vi "Tag FGV.vi"(0 "Operation":T4, 5 "Tag Name":string, 9 "Data":variant, 11 "error in (no error)":errorcluster, 12 "Tag Category":string) -> (2 "Alarm Array":T1[](array[typedef]), 3 "Process Name":string, 4 "Tag Names":string[](array[string]), 6 "Tag Values":dbl[](array[numeric]), 10 "Tag Value":dbl, 13 "Boolean alarm settings":T2, 14 "alarms":T3(array[cluster]) {"value" format="%.2f"; "setpoint" format="%.2f"; "clear time" format="%<%X\n%x>T"; "ack time" format="%<%X\n%x>T"; "set time" format="%<%X\n%x>T"}, 15 "error out":errorcluster)   [LabVIEW 2018, in "Dynamic Shared Variables.lvlib"]
doc: "Handles dynamic tag (shared variable) creation and release as well as alarm configuration and ack."
uses:
  Shared Variables/Dynamic Shared Variables.lvlib
  Tag FGV Operation Enum.ctl
  Numeric Alarm Settings Cluster.ctl
  Utilities/ISO 8601 type.ctl
  Shared Variables/URL Type Enum.ctl
  <vilib>/lvdsc/alarm/Acknowledge Alarms By Instance.vi
  <vilib>/lvdsc/variables/internal/Configure Alarming (Shared Variable, Numeric).vi
  <vilib>/lvdsc/variables/internal/Configure Alarming (Shared Variable, Boolean).vi
  <vilib>/lvdsc/variables/internal/Configure Alarming (Shared Variable, Enable Alarming).vi
  XML Config/XML Config.lvlib
  <vilib>/lvdsc/NI_DSC.lvlib
  <resource>/objmgr/nvio.rc
panel:
  out "Tag Category Array":string[](array[string])
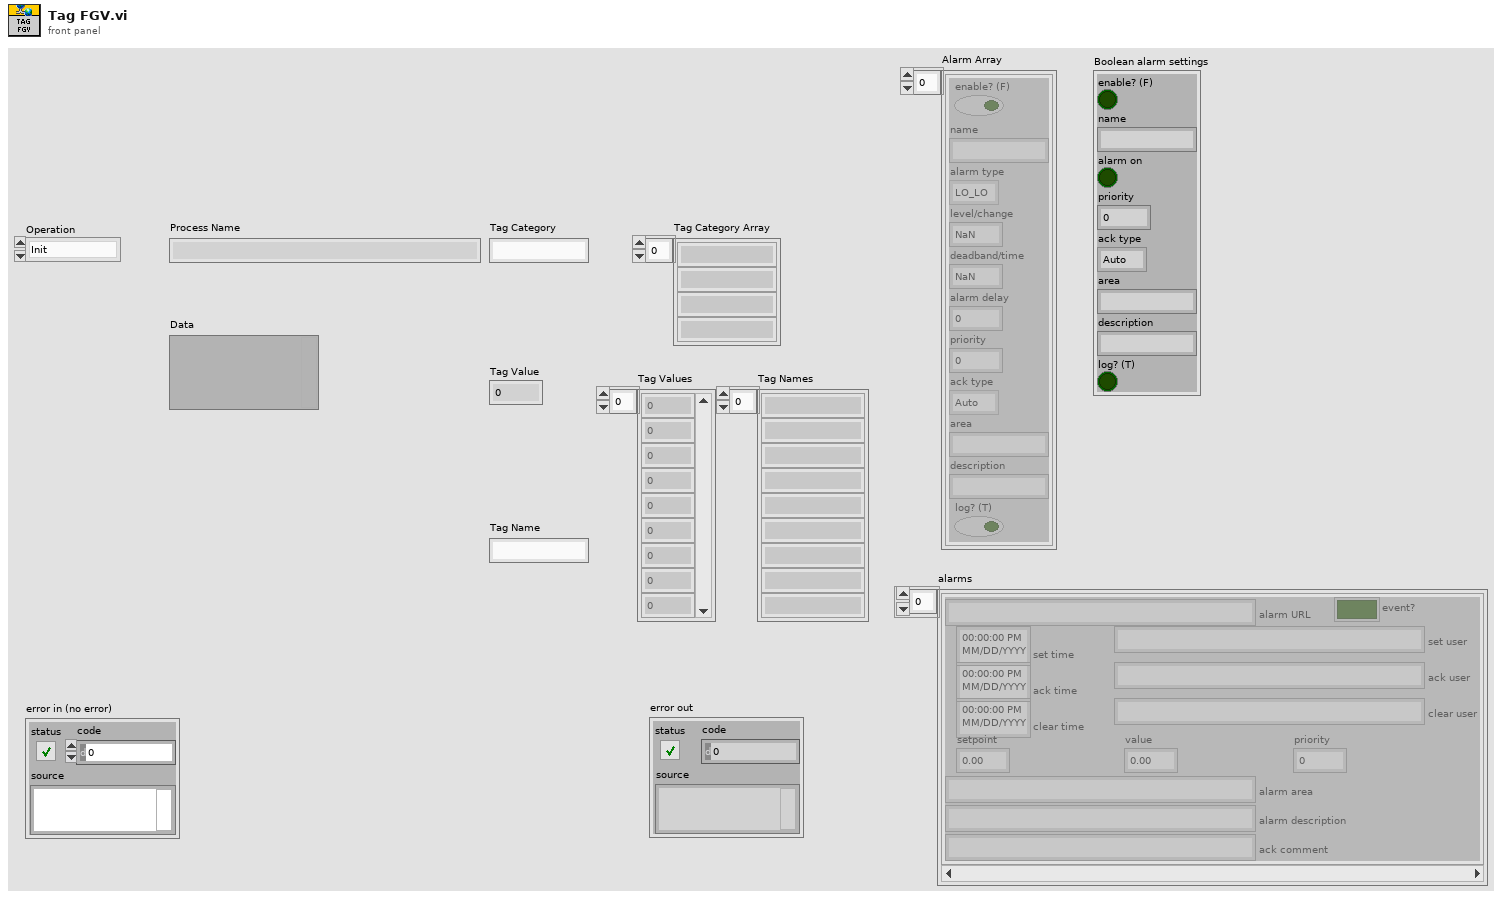
[diagram p1: front panel]
types:
  T1 = typedef "Numeric Alarm Settings Cluster.ctl" = cluster{"enable? (F)":bool, "name":string, "alarm type":enum16{"HI_HI", "HI", "LO", "LO_LO"}, "level/change":dbl, "deadband/time":dbl, "alarm delay":dbl, "priority":u32, "ack type":enum16{"Auto", "User", "None", "Each Occurrence"}, "area":string, "description":string, "log? (T)":bool}
  T2 = cluster{"enable? (F)":bool, "name":string, "alarm on":bool, "priority":u32, "ack type":enum16{"Auto", "User", "None", "Each Occurrence"}, "area":string, "description":string, "log? (T)":bool}
  T3 = cluster{"alarm URL":string, "set time":timestamp, "set user":string, "ack time":timestamp, "ack user":string, "clear time":timestamp, "clear user":string, "setpoint":dbl, "value":dbl, "priority":u32, "alarm area":string, "alarm description":string, "ack comment":string, "event?":bool, "Refnum":u64}[]
  T4 = typedef "Tag FGV Operation Enum.ctl" = enum16{"Init", "Set Notification Queue", "Create Tag", "Commit", "Write Tag (Numeric)", "Write Tag (Boolean)", "Read All Tags", "Read One Tag", "Delete Tag Category", "Set Alarm Parameters (Numeric)", "Set Alarm Parameters (Boolean)", "Enable All Alarms", "Disable All Alarms", "Delete All Tags", "Read Alarms", "Ack Alarm", "Read Alarm Parameters (Numeric)", "Read Alarm Parameters (Boolean)"}
  T5 = typedef "ISO 8601 type.ctl" = enum16{"full ISO 8601 UTC", "basic ISO8601 local", "Windows ISO 8601 UTC", "YYYY-MM-DD UTC", "full ISO 8601 local"}
  T6 = enum32{"u32BitField", "bool", "double", "string", "int8", "uint8", "int16", "uint16", "int32", "uint32", "int64", "uint64", "single", "double waveform", "int16 waveform", "array of boolean", "array of int8", "array of uint8", "array of int16", "array of uint16", "array of int32", "array of uint32", "array of int64", "array of uint64", "array of single", "array of double", "array of double waveform", "array of int16 waveform", "array of string", "variant", "timestamp", "fixed point", "custom"}
  T7 = typedef "Dynamic Shared Variables.lvlib/URL Type Enum.ctl" = enum16{"Tag", "HiHi", "Hi", "Lo", "LoLo", "Tag (Bool)"}
  T8 = cluster{"alarm URL":string, "set time":timestamp, "set user":string, "ack time":timestamp, "ack user":string, "clear time":timestamp, "clear user":string, "setpoint":dbl, "value":dbl, "priority":u32, "alarm area":string, "alarm description":string, "ack comment":string, "event?":bool, "Refnum":u64}
  T9 = enum16{"Auto", "User", "None", "Each Occurrence"}
  T10 = cluster{"enable? (F)":bool, "name":string, "alarm type":enum16{"HI_HI", "HI", "LO", "LO_LO"}, "level/change":dbl, "deadband/time":dbl, "priority":u32, "ack type":enum16{"Auto", "User", "None", "Each Occurrence"}, "area":string, "description":string, "log? (T)":bool}
  T11 = cluster{"enable? (F)":bool, "name":string, "alarm on":bool, "priority":u32, "ack type":enum16{"Auto", "User", "None", "Each Occurrence"}, "area":string, "description":string, "log? (T)":bool}[]
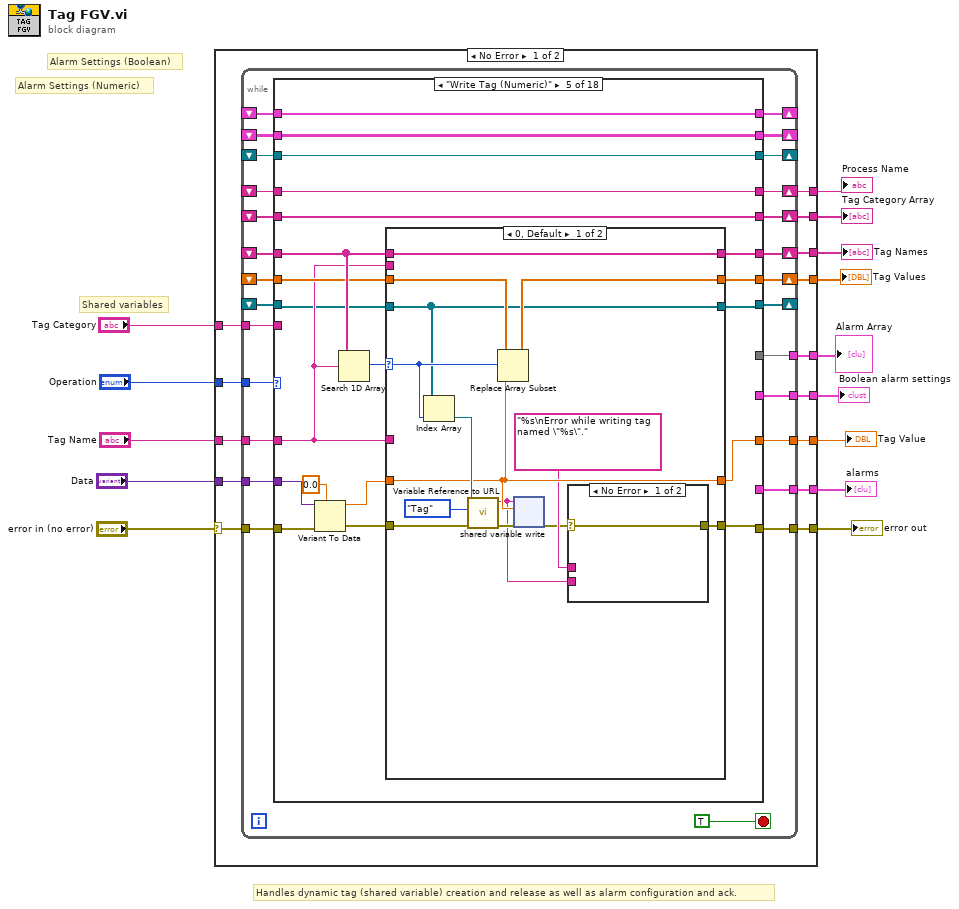
[diagram p0: block diagram]
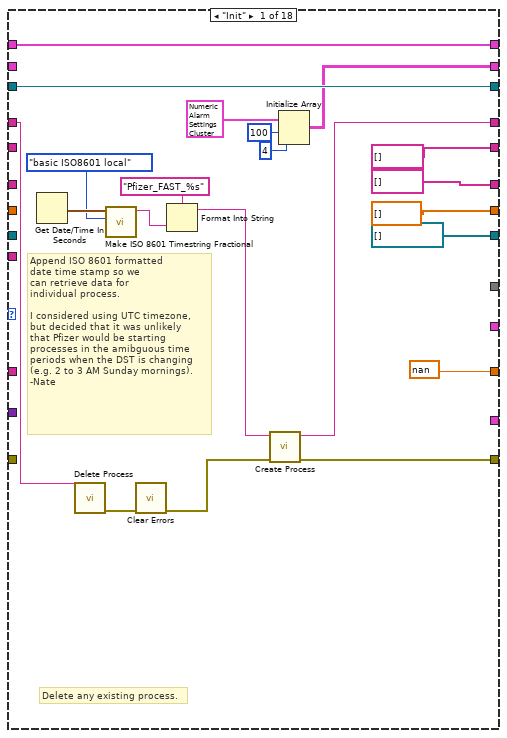
[diagram p2: hidden frame]
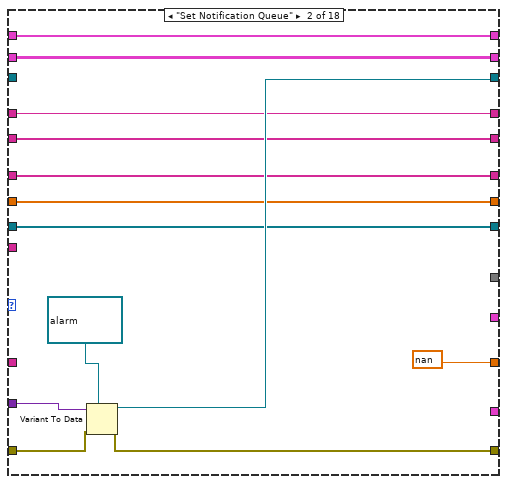
[diagram p3: hidden frame]
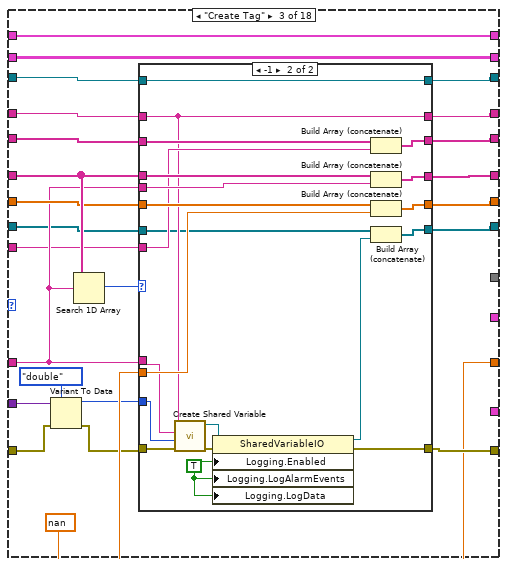
[diagram p4: hidden frame]
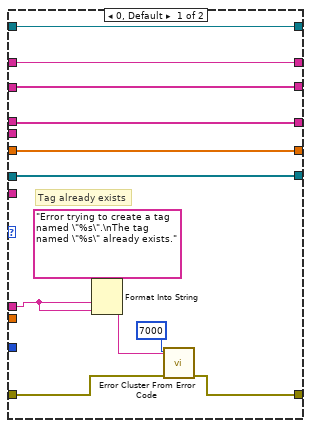
[diagram p5: hidden frame]
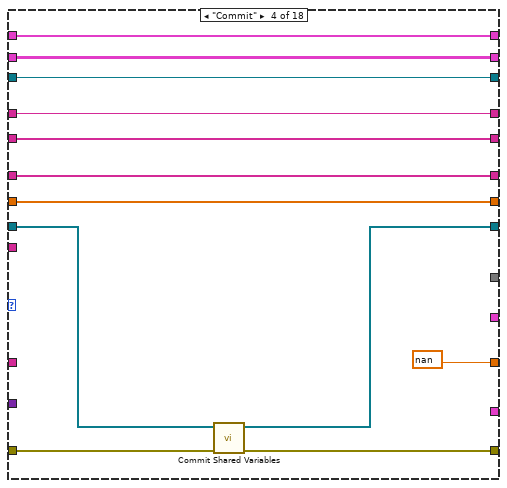
[diagram p6: hidden frame]
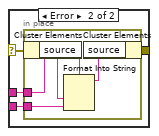
[diagram p7: hidden frame]
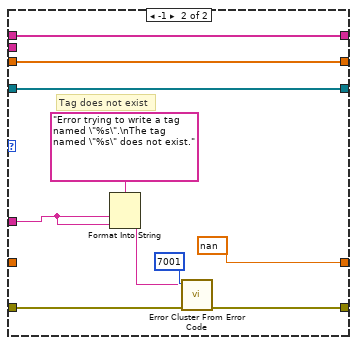
[diagram p8: hidden frame]
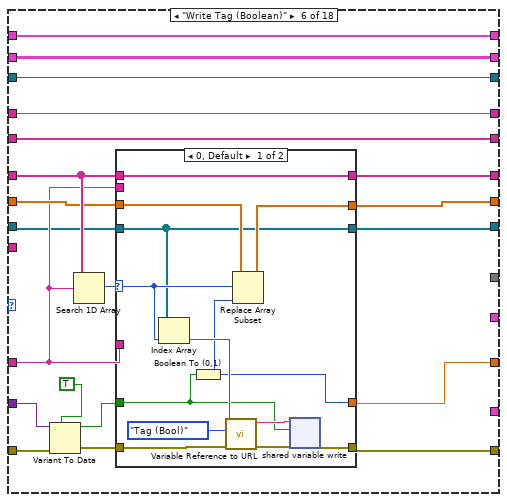
[diagram p9: hidden frame]
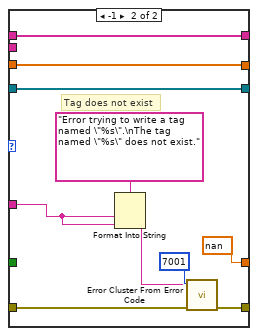
[diagram p10: hidden frame]
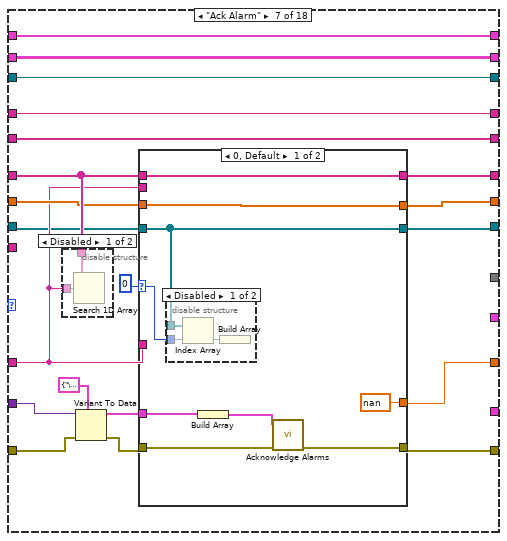
[diagram p11: hidden frame]
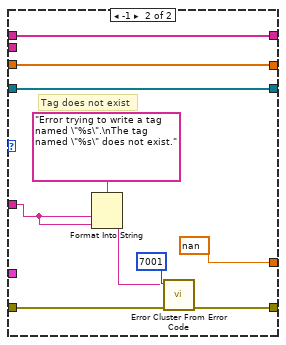
[diagram p14: hidden frame]
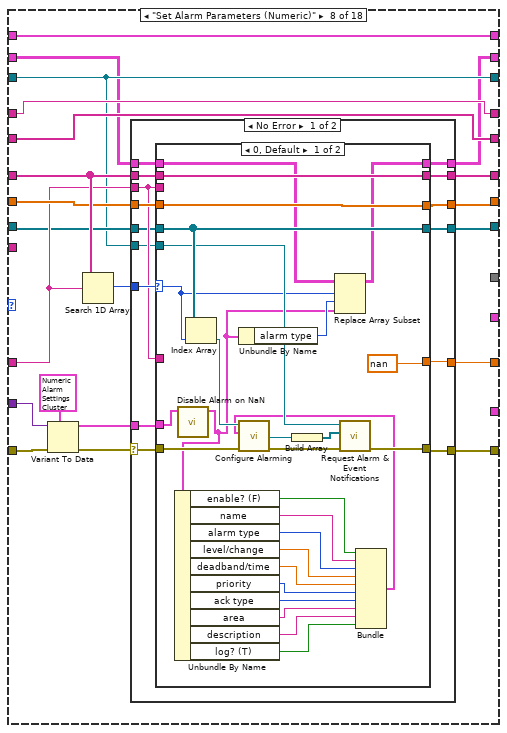
[diagram p15: hidden frame]
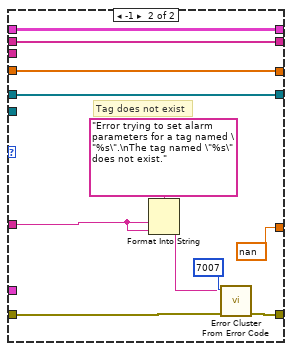
[diagram p16: hidden frame]
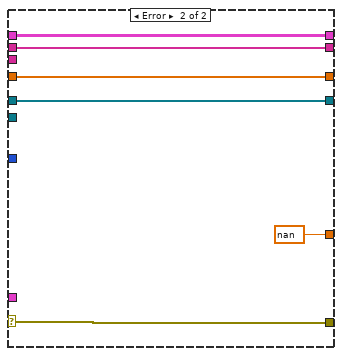
[diagram p17: hidden frame]
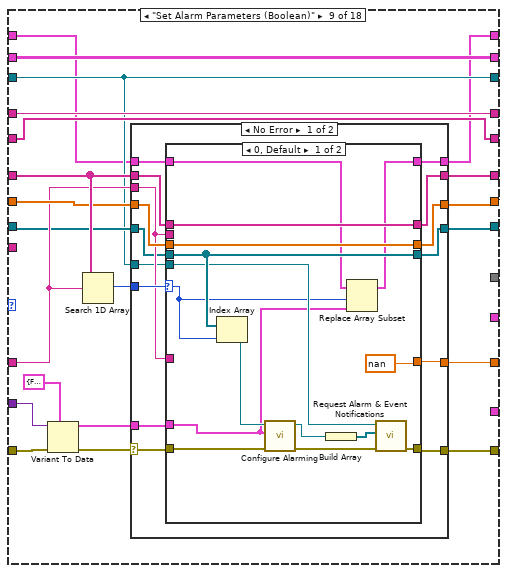
[diagram p18: hidden frame]
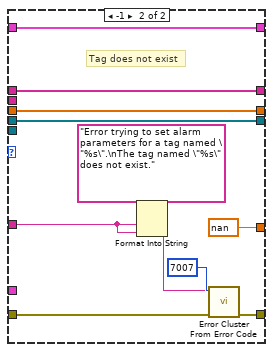
[diagram p19: hidden frame]
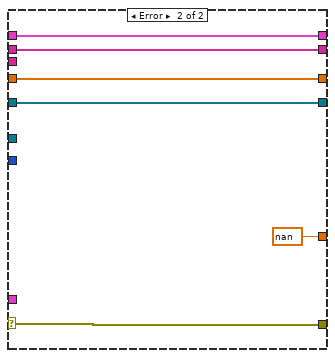
[diagram p20: hidden frame]
diagram:
  # "Alarm Settings (Boolean)"
  # "Alarm Settings (Numeric)"
  # "Handles dynamic tag (shared variable) creation and release as well as alarm configuration and ack."
  # "Shared variables"
  n1 = case shown="No Error" "error in (no error)" {
    selector: "error in (no error)" -> [w25 w626]
    tunnel: [w24 w626] -> w13
    tunnel: "Operation" -> [w28 _]
    tunnel: "Tag Name" -> [w27 _]
    tunnel: "Data" -> [w26 _]
    tunnel: [w23 _] -> w9
    tunnel: [w22 _] -> w8
    tunnel: [w21 nan ("Tag Value (NaN)")] -> w7
    tunnel: "Tag Category" -> [w20 _]
    tunnel: [w19 _] -> w5
    tunnel: [w18 _] -> w4
    tunnel: [w17 _] -> w3
    tunnel: [w16 _] -> w2
    tunnel: [w15 _] -> w1
    frame No Error {
      n2 = while {
        tunnel: w28 -> [w54]
        shift-right: [w52] -> w22
        shift-left: _ -> [w51]
        shift-right: [w53] -> w23
        shift-left: _ -> [w49]
        tunnel: w27 -> [w50]
        tunnel: w26 -> [w48]
        tunnel: w25 -> [w47]
        tunnel: [w45] -> w24
        tunnel: [w46] -> w21
        shift-right: [w44] -> w19
        shift-left: _ -> [w43]
        tunnel: w20 -> [w42]
        shift-right: [w41] -> w17
        shift-left: _ -> [w40]
        shift-right: [w39] -> _
        shift-left: _ -> [w38]
        tunnel: [w37] -> w18
        shift-right: [w36] -> _
        shift-left: _ -> [w35]
        shift-right: [w34] -> _
        shift-left: _ -> [w33]
        shift-right: [w32] -> _
        shift-left: _ -> [w31]
        tunnel: [w30] -> w16
        tunnel: [w29] -> w15
        stop <- TRUE stop-if-true
        n3 = case shown="\"Write Tag (Numeric)\"" w54 {
          tunnel: [dbl[] [] ("Tag Values") w84 w109 w157 w174 w227 w271 w315 w396 w457 w468 w487 w503 w519 dbl[] [] ("Tag Values") w567 w584 w611] -> w53
          tunnel: [string[] [] ("Tag Names") w82 w111 w158 w176 w229 w273 w317 w398 w456 w470 w488 w504 w521 w550 w566 w580 w607] -> w52
          tunnel: w51 -> [_ w82 w112 w158 w177 w230 w274 w318 w399 w456 w470 w488 w504 w522 _ w566 w580 w607]
          tunnel: w50 -> [_ _ w108 _ w173 w226 w270 w314 w395 _ w469 _ _ w526 _ _ w575 w601]
          tunnel: w49 -> [_ w84 w110 w157 w175 w228 w272 w316 w397 w457 w468 w487 w503 w520 _ w567 w584 w611]
          tunnel: w48 -> [_ w88 w98 _ w162 w215 w263 w306 w387 _ _ _ _ _ _ _ _ _]
          tunnel: w47 -> [_ w86 w96 w150 w165 w218 w261 w304 w385 w455 w464 w477 w493 w509 w545 w571 w578 w605]
          tunnel: [w72 w85 w107 w156 w172 w225 w269 w313 w394 w455 w465 w482 w498 w515 w547 w570 w577 w604] -> w45
          tunnel: [nan ("Tag Value (NaN)") nan ("Tag Value (NaN)") w99 nan ("Tag Value (NaN)") w171 w224 w268 w312 w393 nan ("Tag Value (NaN)") w467 nan nan nan ("Tag Value (NaN)") nan ("Tag Value (NaN)") nan ("Tag Value (NaN)") nan ("Tag Value (NaN)") nan ("Tag Value (NaN)")] -> w46
          tunnel: [string[] [] ("Tag Names") w81 w104 w155 w170 w223 w267 w311 w392 w453 w463 w486 w502 w523 w550 w565 w585 w612] -> w44
          tunnel: w43 -> [_ w81 w106 w155 w170 w223 w267 w311 w392 w453 w463 w486 w502 w524 _ w565 w585 w612]
          tunnel: w42 -> [_ _ w105 _ _ _ _ _ _ _ _ _ _ w525 w553 _ _ _]
          tunnel: [w71 w80 w102 w154 w168 w221 w265 w309 w390 w451 w461 w485 w501 w514 w544 w564 w586 w613] -> w41
          tunnel: w40 -> [w62 w80 w103 w154 w168 w221 w265 w309 w390 w451 w461 w485 w501 w514 w544 w564 w586 w613]
          tunnel: [refnum<k21>[] [] w83 w101 w153 w167 w220 w264 w308 w389 w452 w462 w484 w500 w513 refnum<k21>[] [] w568 w583 w610] -> w39
          tunnel: w38 -> [_ w83 w100 w152 w169 w222 w266 w310 w391 w452 w462 w484 w500 w517 w551 w568 w583 w610]
          tunnel: [_ _ _ _ _ _ _ _ _ _ _ _ _ _ _ w572 _ _] -> w37
          tunnel: [w64 w87 w93 w151 w161 w214 w257 w303 w383 w450 w460 w480 w496 w512 w546 w563 w579 w606] -> w36
          tunnel: w35 -> [w64 _ w92 w151 w161 w214 w257 w303 w383 w450 w460 w480 w496 w512 w546 w563 w579 w606]
          tunnel: [w56 w78 w91 w148 w160 w213 w256 w302 w382 w449 w459 w479 w495 w511 w543 w562 w576 w614] -> w34
          tunnel: w33 -> [_ w78 w91 w148 w160 w213 w256 w301 w382 w449 w459 w479 w495 w511 w543 w562 w576 w614]
          tunnel: [w60 w77 w90 w147 w159 w212 w255 w300 w381 w448 w458 w478 w494 w510 w542 w561 w587 w603] -> w32
          tunnel: w31 -> [w60 w77 w90 w147 w159 w212 w255 w300 w380 w448 w458 w478 w494 w510 w542 w561 w587 w603]
          tunnel: [_ _ _ _ _ _ _ _ _ _ _ _ _ _ _ _ _ w602] -> w30
          tunnel: [_ _ _ _ _ _ _ _ _ _ _ _ _ _ _ _ w574 _] -> w29
          frame "Init" {
            # "Delete any existing process."
            # "Append ISO 8601 formatted\ndate time stamp so we\ncan retrieve data for\nindividual process.\n\nI considered using UTC timezone,\nbut decided that it was unlikely\nthat Pfizer would be starting\nprocesses in the amibguous time\nperiods when the DST is changing\n(e.g. 2 to 3 AM Sunday mornings).\n-Nate"
            n4 = Get Date/Time In Seconds() -> (seconds since 1Jan1904=w69:timestamp)
            n5 = call <vilib>:"Delete Process.vi"("process name"=w62) -> ("error out"=w63:errorcluster)  [unwired: 10 in]
            n6 = call "Make ISO 8601 Timestring Fractional.vi"("ISO 8601 type"=ISO_8601_type."basic ISO8601 local", "Time Stamp"=w69) -> ("ISO 8601 Timestring"=w66:string)  [unwired: 8 in, 1 out]
            n7 = call <vilib>:"Clear Errors.vi"("error in (no error)"=w63) -> ("error out"=w61:errorcluster)  [unwired: 5 in, 1 out]
            n8 = Format Into String(format string="Pfizer_FAST_%s", w66) -> (resulting string=w65:string)  [unwired: 2 in, 1 out]
            n9 = call "Create Process.vi"("error in (no error)"=w61, "process name"=w65) -> ("error out"=w72:errorcluster, "dup process name"=w71:string)  [unwired: 8 in]
            n10 = Initialize Array(T1 {"enable? (F)"=FALSE, "name"="", "alarm type"=enum."LO_LO", "level/change"=nan, "deadband/time"=nan, "alarm delay"=0.0, "priority"=0, "ack type"=enum."Auto", "area"="", "description"="", "log? (T)"=FALSE} ("numeric alarm settings out"), 100 ("dimension size"), 4 ("dimension size")) -> (w56:T1[][])
          }
          frame "Set Notification Queue" {
            n11 = Variant To Data(error in=w86, type=refnum<user-event> refnum ("notification refnum"), Variant=w88) -> (data=w87:refnum<user-event>, error out=w85:errorcluster)
          }
          frame "Create Tag" {
            w99 = nan ("Tag Value (NaN)")
            n12 = Variant To Data(error in=w96, type=T6."double" ("data type"), Variant=w98) -> (data=w94:T6, error out=w97:errorcluster)
            n13 = Search 1D Array(1D array=w112, element=w108) -> (index of element=w113:i32)  [unwired: 1 in]
            n14 = case shown="-1" w113 {
              tunnel: w108 -> [_ w146]
              tunnel: w112 -> [w125 w145]
              tunnel: [w125 w144] -> w111
              tunnel: w110 -> [w124 w143]
              tunnel: w99 -> [_ w142]
              tunnel: [w124 w141] -> w109
              tunnel: w97 -> [w123 w136]
              tunnel: w108 -> [w120 w137]
              tunnel: [w118 w126] -> w107
              tunnel: w106 -> [w117 w140]
              tunnel: w105 -> [_ w139]
              tunnel: [w117 w138] -> w104
              tunnel: w103 -> [w116 w135]
              tunnel: [w116 w135] -> w102
              tunnel: [w115 w134] -> w101
              tunnel: w100 -> [w115 w133]
              tunnel: w94 -> [_ w129]
              tunnel: [w114 w127] -> w93
              tunnel: w92 -> [w114 w127]
              frame 0, Default {
                # "Tag already exists"
                n15 = Format Into String(format string="Error trying to create a tag named \"%s\".\nThe tag named \"%s\" already exists.", w120, w120) -> (resulting string=w119:string)  [unwired: 2 in, 1 out]
                n16 = call <vilib>:"Error Cluster From Error Code.vi"("error in (no error)"=w123, "error message (\"\")"=w119, "error code (0)"=7000) -> ("error out"=w118:errorcluster)  [unwired: 6 in]
              }
              frame -1 {
                w130 = TRUE ("Logging.LogAlarmEvents")
                n17 = call "Create Shared Variable.vi"("error in (no error)"=w136, "data type"=w129, "shared variable name"=w137, "process name out"=w135) -> ("error out"=w132:errorcluster, "shared variable"=w128:refnum<k21>)  [unwired: 6 in]
                n18 = property class="SharedVariableIO"(reference=w128, error in=w132, "Logging.Enabled"=w130, "Logging.LogAlarmEvents"=w130, "Logging.LogData"=w130) -> (reference out=w131:refnum<k21>, error out=w126:errorcluster)
                n19 = Build Array (concatenate)(w140, w139) -> (w138:string[])
                n20 = Build Array (concatenate)(w145, w146) -> (w144:string[])
                n21 = Build Array (concatenate)(w143, w142) -> (w141:dbl[])
                n22 = Build Array (concatenate)(w133, w131) -> (w134:refnum<k21>[])
              }
            }
          }
          frame "Commit" {
            n23 = call <vilib>:"Commit Shared Variables.vi"("error in (no error)"=w150, "shared variables"=w152) -> ("error out"=w156:errorcluster, "shared variables out"=w153:refnum<k21>[])  [unwired: 8 in]
          }
          frame "Write Tag (Numeric)" {
            n24 = Variant To Data(error in=w165, type=0.0, Variant=w162) -> (data=w163:dbl, error out=w164:errorcluster)
            n25 = Search 1D Array(1D array=w177, element=w173) -> (index of element=w178:i32)  [unwired: 1 in]
            n26 = case shown="0, Default" w178 {
              selector: w178 -> [w189 _]
              tunnel: w173 -> [_ _]
              tunnel: w177 -> [w192 w211]
              tunnel: [w192 w211] -> w176
              tunnel: w175 -> [w191 w210]
              tunnel: w163 -> [w186 _]
              tunnel: [w190 w210] -> w174
              tunnel: w164 -> [w185 w209]
              tunnel: w173 -> [_ w206]
              tunnel: [w182 w204] -> w172
              tunnel: [w186 nan ("Tag Value (NaN)")] -> w171
              tunnel: w169 -> [w183 w202]
              tunnel: [w183 w202] -> w167
              frame 0, Default {
                n27 = Index Array(array=w183, index=w189) -> (element=w188:refnum<k21>)
                n28 = call "Variable Reference to URL.vi"("error in (no error)"=w185, "URL type"=URL_Type_Enum."Tag", "variable reference"=w188) -> ("error out"=w184:errorcluster, "URL"=w180:string)  [unwired: 7 in]
                n29 = Replace Array Subset(array=w191, new element=w186, index=w189) -> (w190:dbl[])
                n30 = shared-variable-write(w180, w184, w186) -> (w179:errorcluster)  [unwired: 1 out]
                n31 = case shown="No Error" w179 {
                  selector: w179 -> [w193 w196]
                  tunnel: [w193 w195] -> w182
                  tunnel: "%s\nError while writing tag named \"%s\"." ("format string") -> [_ w194]
                  tunnel: w180 -> [_ w197]
                  frame No Error {
                  }
                  frame Error {
                    n32 = in-place {
                      in-place-border: w197 -> [w201]
                      in-place-border: w194 -> [w198]
                      n33 = in-place-cluster #1(w196) -> ("source"=w199:string)
                      n34 = Format Into String(format string=w198, w199, w201) -> (resulting string=w200:string)  [unwired: 2 in, 1 out]
                      n35 = in-place-cluster #1("source"=w200) -> (w195:errorcluster)
                    }
                  }
                }
              }
              frame -1 {
                # "Tag does not exist"
                n36 = Format Into String(format string="Error trying to write a tag named \"%s\".\nThe tag named \"%s\" does not exist.", w206, w206) -> (resulting string=w205:string)  [unwired: 2 in, 1 out]
                n37 = call <vilib>:"Error Cluster From Error Code.vi"("error in (no error)"=w209, "error message (\"\")"=w205, "error code (0)"=7001) -> ("error out"=w204:errorcluster)  [unwired: 6 in]
              }
            }
          }
          frame "Write Tag (Boolean)" {
            n38 = Variant To Data(error in=w218, type=TRUE, Variant=w215) -> (data=w216:bool, error out=w217:errorcluster)
            n39 = Search 1D Array(1D array=w230, element=w226) -> (index of element=w231:i32)  [unwired: 1 in]
            n40 = case shown="0, Default" w231 {
              selector: w231 -> [w241 _]
              tunnel: w226 -> [_ _]
              tunnel: w230 -> [w244 w254]
              tunnel: [w244 w254] -> w229
              tunnel: w228 -> [w243 w253]
              tunnel: w216 -> [w233 _]
              tunnel: [w242 w253] -> w227
              tunnel: w217 -> [w237 w252]
              tunnel: w226 -> [_ w249]
              tunnel: [w235 w247] -> w225
              tunnel: [w232 nan ("Tag Value (NaN)")] -> w224
              tunnel: w222 -> [w234 w245]
              tunnel: [w234 w245] -> w220
              frame 0, Default {
                n41 = Index Array(array=w234, index=w241) -> (element=w240:refnum<k21>)
                n42 = Boolean To (0,1)(Boolean=w233) -> (0, 1=w232:i16)
                n43 = call "Variable Reference to URL.vi"("error in (no error)"=w237, "URL type"=URL_Type_Enum."Tag (Bool)", "variable reference"=w240) -> ("error out"=w236:errorcluster, "URL"=w238:string)  [unwired: 7 in]
                n44 = Replace Array Subset(array=w243, new element=w232, index=w241) -> (w242:dbl[])
                n45 = shared-variable-write(w238, w236, w233) -> (w235:errorcluster)  [unwired: 1 out]
              }
              frame -1 {
                # "Tag does not exist"
                n46 = Format Into String(format string="Error trying to write a tag named \"%s\".\nThe tag named \"%s\" does not exist.", w249, w249) -> (resulting string=w248:string)  [unwired: 2 in, 1 out]
                n47 = call <vilib>:"Error Cluster From Error Code.vi"("error in (no error)"=w252, "error message (\"\")"=w248, "error code (0)"=7001) -> ("error out"=w247:errorcluster)  [unwired: 6 in]
              }
            }
          }
          frame "Ack Alarm" {
            n48 = disable-structure shown="Disabled" {
              disable-tunnel: w274 -> [w276 _]
              disable-tunnel: w270 -> [w275 _]
              frame Disabled {
                n49 = Search 1D Array(1D array=w276, element=w275) -> ()  [unwired: 1 in, 1 out]
              }
              frame Enabled {
              }
            }
            n50 = Variant To Data(error in=w261, type=T8 {"alarm URL"="\\\\Nate-VM-LV2018\\Pfizer FAST\\TT1.Alarms.TT1:LoLo", "set time"=timestamp(3634824876.5239263 s since 1904-01-01), "set user"="(Nobody)", "ack time"=timestamp(-9223372036854775808 s since 1904-01-01), "ack user"="", "clear time"=timestamp(-9223372036854775808 s since 1904-01-01), "clear user"="", "setpoint"=20.0, "value"=19.923748781652513, "priority"=100, "alarm area"="", "alarm description"="", "ack comment"="", "event?"=FALSE, "Refnum"=216172782113783885} ("Alarm"), Variant=w263) -> (data=w260:T8, error out=w262:errorcluster)
            n51 = case shown="0, Default" 0 ("index of element") {
              selector: 0 ("index of element") -> [w284 _]
              tunnel: w270 -> [_ _]
              tunnel: w274 -> [w285 w298]
              tunnel: [w285 w298] -> w273
              tunnel: w272 -> [w282 w297]
              tunnel: [w282 w297] -> w271
              tunnel: w262 -> [w280 w296]
              tunnel: w270 -> [_ w293]
              tunnel: [w279 w291] -> w269
              tunnel: [nan ("Tag Value (NaN)") nan ("Tag Value (NaN)")] -> w268
              tunnel: w266 -> [w283 w289]
              tunnel: [w283 w289] -> w264
              tunnel: w260 -> [w278 _]
              frame 0, Default {
                n52 = disable-structure shown="Disabled" {
                  disable-tunnel: w284 -> [w288 _]
                  disable-tunnel: w283 -> [w287 _]
                  frame Disabled {
                    n53 = Index Array(array=w287, index=w288) -> (element=w286:refnum<k21>)
                    n54 = Build Array(w286) -> ()  [unwired: 1 out]
                  }
                  frame Enabled {
                  }
                }
                n55 = Build Array(w278) -> (w277:T3)
                n56 = call-poly <vilib>:"Acknowledge Alarms.vi"("error in (no error)"=w280, "alarms"=w277) -> ("error out"=w279:errorcluster)  [unwired: 9 in]
              }
              frame -1 {
                # "Tag does not exist"
                n57 = Format Into String(format string="Error trying to write a tag named \"%s\".\nThe tag named \"%s\" does not exist.", w293, w293) -> (resulting string=w292:string)  [unwired: 2 in, 1 out]
                n58 = call <vilib>:"Error Cluster From Error Code.vi"("error in (no error)"=w296, "error message (\"\")"=w292, "error code (0)"=7001) -> ("error out"=w291:errorcluster)  [unwired: 6 in]
              }
            }
          }
          frame "Set Alarm Parameters (Numeric)" {
            n59 = Variant To Data(error in=w304, type=T1 {"enable? (F)"=FALSE, "name"="", "alarm type"=enum."LO_LO", "level/change"=nan, "deadband/time"=nan, "alarm delay"=0.0, "priority"=0, "ack type"=enum."Auto", "area"="", "description"="", "log? (T)"=FALSE} ("numeric alarm settings out"), Variant=w306) -> (data=w307:T1, error out=w305:errorcluster)
            n60 = Search 1D Array(1D array=w318, element=w314) -> (index of element=w319:i32)  [unwired: 1 in]
            n61 = case shown="No Error" w305 {
              selector: w305 -> [w323 w375]
              tunnel: w319 -> [w334 _]
              tunnel: w318 -> [w333 w377]
              tunnel: [w332 w377] -> w317
              tunnel: w316 -> [w331 w378]
              tunnel: w307 -> [w330 _]
              tunnel: [w329 w378] -> w315
              tunnel: w314 -> [w328 _]
              tunnel: [w327 w375] -> w313
              tunnel: [w326 nan ("Tag Value (NaN)")] -> w312
              tunnel: w310 -> [w325 w379]
              tunnel: [w324 w379] -> w308
              tunnel: w303 -> [w322 _]
              tunnel: [w321 w374] -> w302
              tunnel: w301 -> [w320 w374]
              frame No Error {
                n62 = case shown="0, Default" w334 {
                  selector: w334 -> [w350 _]
                  tunnel: w328 -> [_ _]
                  tunnel: w333 -> [w362 w373]
                  tunnel: [w362 w373] -> w332
                  tunnel: w331 -> [w357 w372]
                  tunnel: w330 -> [w356 _]
                  tunnel: [w357 w372] -> w329
                  tunnel: w323 -> [w359 w371]
                  tunnel: w328 -> [_ w364]
                  tunnel: [w351 w367] -> w327
                  tunnel: [nan nan ("Tag Value (NaN)")] -> w326
                  tunnel: w325 -> [w361 w365]
                  tunnel: [w361 w365] -> w324
                  tunnel: w322 -> [w353 _]
                  tunnel: [w349 w363] -> w321
                  tunnel: w320 -> [w348 w363]
                  frame 0, Default {
                    n63 = call "Disable Alarm on NaN.vi"("numeric alarm settings in"=w356) -> ("numeric alarm settings out"=w346:T1)  [unwired: 10 in]
                    n64 = Unbundle By Name(w346) -> ("enable? (F)"=w345:bool, "name"=w344:string, "alarm type"=w343:enum16{"HI_HI", "HI", "LO", "LO_LO"}, "level/change"=w342:dbl, "deadband/time"=w341:dbl, "priority"=w340:u32, "ack type"=w339:T9, "area"=w338:string, "description"=w337:string, "log? (T)"=w336:bool)
                    n65 = Index Array(array=w361, index=w350) -> (element=w360:refnum<k21>)
                    n66 = Unbundle By Name(w346) -> ("alarm type"=w347:enum16{"HI_HI", "HI", "LO", "LO_LO"})
                    n67 = Replace Array Subset(array=w348, new element=w346, index (row)=w350, index (col)=w347) -> (w349:T1[][])
                    n68 = Bundle("enable? (F)"=w345, "name"=w344, "alarm type"=w343, "level/change"=w342, "deadband/time"=w341, "priority"=w340, "ack type"=w339, "area"=w338, "description"=w337, "log? (T)"=w336) -> (w335:T10)  [unwired: 1 in]
                    n69 = call-poly <vilib>:"Configure Alarming.vi"("error in (no error)"=w359, "numeric alarm settings"=w335, "variable reference in"=w360) -> ("error out"=w352:errorcluster, "variable reference out"=w354:refnum<k21>)  [unwired: 7 in]
                    n70 = Build Array(w354) -> (w355:refnum<k21>[])
                    n71 = call <vilib>:"Request Alarm & Event Notifications.vi"("error in (no error)"=w352, "shared variables"=w355, "notification refnum"=w353) -> ("error out"=w351:errorcluster)  [unwired: 6 in, 2 out]
                  }
                  frame -1 {
                    # "Tag does not exist"
                    n72 = Format Into String(format string="Error trying to set alarm parameters for a tag named \"%s\".\nThe tag named \"%s\" does not exist.", w364, w364) -> (resulting string=w368:string)  [unwired: 2 in, 1 out]
                    n73 = call <vilib>:"Error Cluster From Error Code.vi"("error in (no error)"=w371, "error message (\"\")"=w368, "error code (0)"=7007) -> ("error out"=w367:errorcluster)  [unwired: 6 in]
                  }
                }
              }
              frame Error {
              }
            }
          }
          frame "Set Alarm Parameters (Boolean)" {
            n74 = Variant To Data(error in=w385, type=T2 {"enable? (F)"=FALSE, "name"="Boolean", "alarm on"=TRUE, "priority"=1, "ack type"=enum."Auto", "area"="", "description"="", "log? (T)"=TRUE} ("Boolean alarm settings"), Variant=w387) -> (data=w388:T2, error out=w386:errorcluster)
            n75 = Search 1D Array(1D array=w399, element=w395) -> (index of element=w400:i32)  [unwired: 1 in]
            n76 = case shown="No Error" w386 {
              selector: w386 -> [w404 w443]
              tunnel: w400 -> [w415 _]
              tunnel: w399 -> [w414 w445]
              tunnel: [w413 w445] -> w398
              tunnel: w397 -> [w412 w446]
              tunnel: w388 -> [w411 _]
              tunnel: [w410 w446] -> w396
              tunnel: w395 -> [w409 _]
              tunnel: [w408 w443] -> w394
              tunnel: [w407 nan ("Tag Value (NaN)")] -> w393
              tunnel: w391 -> [w406 w447]
              tunnel: [w405 w447] -> w389
              tunnel: w383 -> [w403 _]
              tunnel: [w402 w442] -> w381
              tunnel: w380 -> [w401 w442]
              frame No Error {
                n77 = case shown="0, Default" w415 {
                  selector: w415 -> [w419 _]
                  tunnel: w409 -> [_ _]
                  tunnel: w414 -> [w430 w441]
                  tunnel: [w430 w441] -> w413
                  tunnel: w412 -> [w425 w440]
                  tunnel: w411 -> [w417 _]
                  tunnel: [w425 w440] -> w410
                  tunnel: w404 -> [w427 w439]
                  tunnel: w409 -> [_ w432]
                  tunnel: [w420 w435] -> w408
                  tunnel: [nan nan ("Tag Value (NaN)")] -> w407
                  tunnel: w406 -> [w429 w433]
                  tunnel: [w429 w433] -> w405
                  tunnel: w403 -> [w423 _]
                  tunnel: [w418 w431] -> w402
                  tunnel: w401 -> [w416 w431]
                  frame 0, Default {
                    n78 = Index Array(array=w429, index=w419) -> (element=w428:refnum<k21>)
                    n79 = call-poly <vilib>:"Configure Alarming.vi"("error in (no error)"=w427, "Boolean alarm settings"=w417, "variable reference in"=w428) -> ("error out"=w421:errorcluster, "variable reference out"=w422:refnum<k21>)  [unwired: 7 in]
                    n80 = Build Array(w422) -> (w424:refnum<k21>[])
                    n81 = Replace Array Subset(array=w416, new element=w417, index=w419) -> (w418:T11)
                    n82 = call <vilib>:"Request Alarm & Event Notifications.vi"("error in (no error)"=w421, "shared variables"=w424, "notification refnum"=w423) -> ("error out"=w420:errorcluster)  [unwired: 6 in, 2 out]
                  }
                  frame -1 {
                    # "Tag does not exist"
                    n83 = Format Into String(format string="Error trying to set alarm parameters for a tag named \"%s\".\nThe tag named \"%s\" does not exist.", w432, w432) -> (resulting string=w436:string)  [unwired: 2 in, 1 out]
                    n84 = call <vilib>:"Error Cluster From Error Code.vi"("error in (no error)"=w439, "error message (\"\")"=w436, "error code (0)"=7007) -> ("error out"=w435:errorcluster)  [unwired: 6 in]
                  }
                }
              }
              frame Error {
              }
            }
          }
          frame "Read All Tags" {
          }
          frame "Read One Tag" {
            n85 = Search 1D Array(1D array=w470, element=w469) -> (index of element=w466:i32)  [unwired: 1 in]
            n86 = case shown="-1" w466 {
              selector: w466 -> [_ w474]
              tunnel: w468 -> [_ w476]
              tunnel: [nan ("Tag Value (NaN)") w475] -> w467
              tunnel: [errorcluster {"status"=TRUE, "code"=7002, "source"="Tag Name not found in Tag Names in Tag FGV.vi"} ("error IO") w473] -> w465
              tunnel: w464 -> [_ w473]
              frame -1 {
              }
              frame Default {
                n87 = Index Array(array=w476, index=w474) -> (element=w475:dbl)
              }
            }
          }
          frame "Enable All Alarms" {
            n88 = for {
              tunnel: w484 -> [w491] mode=indexing
              tunnel: w477 -> [w490]
              tunnel: [w489] -> w483 mode=indexing
              n89 = call-poly <vilib>:"Configure Alarming.vi"("error in (no error)"=w490, "enable? (F)"=TRUE, "variable reference in"=w491) -> ("error out"=w489:errorcluster)  [unwired: 7 in, 1 out]
            }
            n90 = Merge Errors(w477, w483) -> (w482:errorcluster)
          }
          frame "Disable All Alarms" {
            n91 = for {
              tunnel: w500 -> [w507] mode=indexing
              tunnel: w493 -> [w506]
              tunnel: [w505] -> w499 mode=indexing
              n92 = call-poly <vilib>:"Configure Alarming.vi"("error in (no error)"=w506, "enable? (F)"=FALSE, "variable reference in"=w507) -> ("error out"=w505:errorcluster)  [unwired: 7 in, 1 out]
            }
            n93 = Merge Errors(w493, w499) -> (w498:errorcluster)
          }
          frame "Delete Tag Category" {
            # "Delete all tags matching the tag category. This is to support when\na user picks a new DAQmx task, and the channels (i.e. tags) of the\nnew task will replace all the channels (i.e. tags) of the old task.\n\nThus this case is used to delete all the DAQ tags."
            n94 = for {
              tunnel: w526 -> [_]
              tunnel: w524 -> [w533] mode=indexing
              tunnel: w522 -> [w532] mode=indexing
              tunnel: w520 -> [w531] mode=indexing
              tunnel: w525 -> [w534]
              tunnel: [w533] -> w523 mode=indexing if=w527
              tunnel: [w532] -> w521 mode=indexing if=w527
              tunnel: [w531] -> w519 mode=indexing if=w527
              tunnel: w517 -> [w528] mode=indexing
              tunnel: w509 -> [w530]
              tunnel: [w529] -> w516 mode=indexing
              tunnel: [w528] -> w513 mode=indexing if=w527
              n95 = Not Equal?(x=w533, y=w534) -> (x != y?=w527:bool)
              n96 = case shown="False" w527 {
                tunnel: w528 -> [w537 _]
                tunnel: w530 -> [w536 w538]
                tunnel: [w535 w538] -> w529
                frame False {
                  n97 = call <vilib>:"Delete Shared Variable.vi"("error in (no error)"=w536, "shared variable"=w537) -> ("error out"=w535:errorcluster)  [unwired: 9 in]
                }
                frame True {
                }
              }
            }
            n98 = Merge Errors(w509, w516) -> (w515:errorcluster)
          }
          frame "Delete All Tags" {
            w550 = string[] [] ("Tag Names")
            # "Delete all tags matching the tag category. This is to support when\na user picks a new DAQmx task, and the channels (i.e. tags) of the\nnew task will replace all the channels (i.e. tags) of the old task.\n\nThus this case is used to delete all the DAQ tags."
            n99 = call <vilib>:"Disable Alarm & Event Notifications.vi"("error in (no error)"=w545, "notification refnum"=w546) -> ("error out"=w540:errorcluster)  [unwired: 9 in]
            n100 = for {
              tunnel: w553 -> [_]
              tunnel: w551 -> [w558] mode=indexing
              tunnel: w540 -> [w560]
              tunnel: [w559] -> w541 mode=indexing
              n101 = call <vilib>:"Delete Shared Variable.vi"("error in (no error)"=w560, "shared variable"=w558) -> ("error out"=w559:errorcluster)  [unwired: 9 in]
            }
            n102 = Merge Errors(w540, w541) -> (w539:errorcluster)
            n103 = flat-sequence {
              tunnel: [w556] -> w547
              tunnel: w544 -> [w555]
              tunnel: w539 -> [w554]
              frame #0 {
                n104 = call <vilib>:"Delete Process.vi"("error in (no error)"=w554, "process name"=w555) -> ("error out"=w557:errorcluster)  [unwired: 9 in]
                n105 = call <vilib>:"Clear Errors.vi"("error in (no error)"=w557) -> ("error out"=w556:errorcluster)  [unwired: 5 in, 1 out]
              }
            }
          }
          frame "Read Alarms" {
            n106 = call <vilib>:"Read Alarms.vi"("error in (no error)"=w571, "timeout (s)"=1, "shared variables"=w568) -> ("error out"=w570:errorcluster, "alarms"=w572:T3)  [unwired: 7 in]
          }
          frame "Read Alarm Parameters (Numeric)" {
            n107 = Search 1D Array(1D array=w580, element=w575) -> (index of element=w581:i32)  [unwired: 1 in]
            n108 = case shown="-1" w581 {
              selector: w581 -> [w589 _]
              tunnel: [w594 w597] -> w577
              tunnel: w578 -> [w594 _]
              tunnel: w576 -> [w593 _]
              tunnel: [w588 T1[] [{"enable? (F)"=FALSE, "name"="", "alarm type"=enum."LO_LO", "level/change"=nan, "deadband/time"=nan, "alarm delay"=0.0, "priority"=0, "ack type"=enum."Auto", "area"="", "description"="", "log? (T)"=FALSE}]] -> w574
              tunnel: w575 -> [_ w596]
              frame 0, Default {
                n109 = Index Array(array=w593, index (row)=w589) -> (element=w592:T1[])  [unwired: 1 in]
                n110 = Array Subset(array=w592, index=0, length=4) -> (w588:T1[])
              }
              frame -1 {
                # "Tag does not exist"
                n111 = Format Into String(format string="Error trying to retrieve alarm parameters for a tag named \"%s\".\nThe tag named \"%s\" does not exist.", w596, w596) -> (resulting string=w598:string)  [unwired: 2 in, 1 out]
                n112 = call <vilib>:"Error Cluster From Error Code.vi"("error message (\"\")"=w598, "error code (0)"=7007) -> ("error out"=w597:errorcluster)  [unwired: 7 in]
              }
            }
          }
          frame "Read Alarm Parameters (Boolean)" {
            n113 = Search 1D Array(1D array=w607, element=w601) -> (index of element=w608:i32)  [unwired: 1 in]
            n114 = case shown="0, Default" w608 {
              selector: w608 -> [w616 _]
              tunnel: [w618 w621] -> w604
              tunnel: w605 -> [w618 _]
              tunnel: w603 -> [w617 _]
              tunnel: [w615 T2 {"enable? (F)"=FALSE, "name"="", "alarm on"=FALSE, "priority"=0, "ack type"=enum."Auto", "area"="", "description"="", "log? (T)"=FALSE} ("Boolean alarm settings")] -> w602
              tunnel: w601 -> [_ w619]
              frame 0, Default {
                n115 = Index Array(array=w617, index=w616) -> (element=w615:T2)
              }
              frame -1 {
                # "Tag does not exist"
                n116 = Format Into String(format string="Error trying to retrieve alarm parameters for a tag named \"%s\".\nThe tag named \"%s\" does not exist.", w619, w619) -> (resulting string=w622:string)  [unwired: 2 in, 1 out]
                n117 = call <vilib>:"Error Cluster From Error Code.vi"("error message (\"\")"=w622, "error code (0)"=7007) -> ("error out"=w621:errorcluster)  [unwired: 7 in]
              }
            }
          }
        }
      }
    }
    frame Error {
    }
  }
  "error out" <- w13
  "Tag Names" <- w8
  "Tag Values" <- w9
  "Tag Value" <- w7
  "Tag Category Array" <- w5
  "alarms" <- w4
  "Process Name" <- w3
  "Boolean alarm settings" <- w2
  "Alarm Array" <- w1
